vi "GetSolenoidRefnum.vi"() -> (3 "GetRefnumSolenoid":string)   [LabVIEW 2016, in "Gear Manipulator.lvclass"]
uses:
  Gear Manipulator.lvclass
  Gear Manipulator.lvclass/Gear Manipulator.ctl
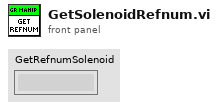
[diagram p1: front panel]
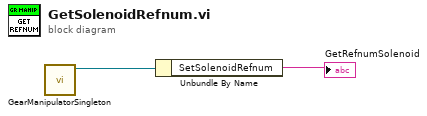
[diagram p0: block diagram]
diagram:
  n1 = call "GearManipulatorSingleton.vi"() -> ("Gear Manipulator.lvclass"=w2:refnum<class "Gear Manipulator.lvclass">)  [unwired: 10 in, 1 out]
  n2 = Unbundle By Name(w2) -> ("SetSolenoidRefnum"=→"GetRefnumSolenoid":string)
